vi "Filter Linearity Results.vi"(8 "error in (no error)":errorcluster, 10 "SensorID":i32, 11 "Linearity Results":T1[](array[typedef])) -> (0 "error out":errorcluster, 3 "Filtered Linearity Results":T1[](array[typedef]))   [LabVIEW 2026, in "Analysis.lvlib"]
uses:
  Analysis.lvlib
  Linearity Result.ctl
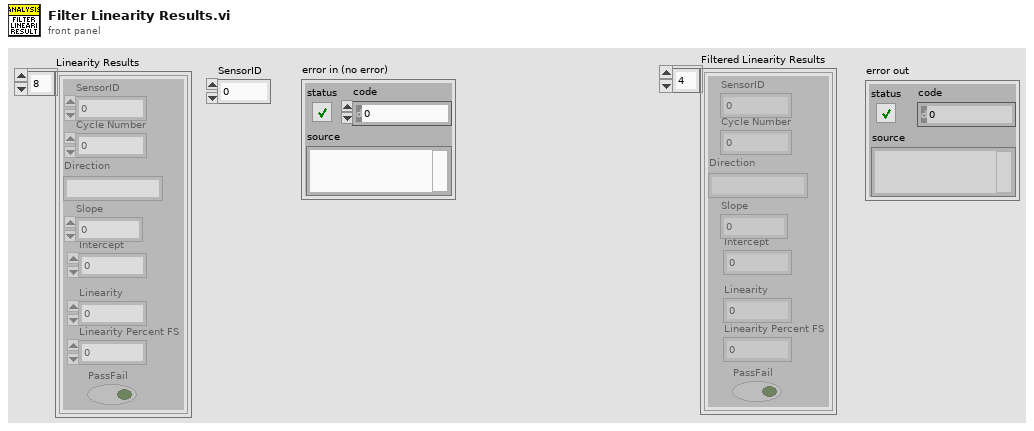
[diagram p1: front panel]
types:
  T1 = typedef "Analysis.lvlib/Linearity Result.ctl" = cluster{"Slope":dbl, "Intercept":dbl, "Cycle Number":i32, "SensorID":i32, "Linearity":dbl, "Linearity Percent FS":dbl, "Direction":string, "PassFail":bool}
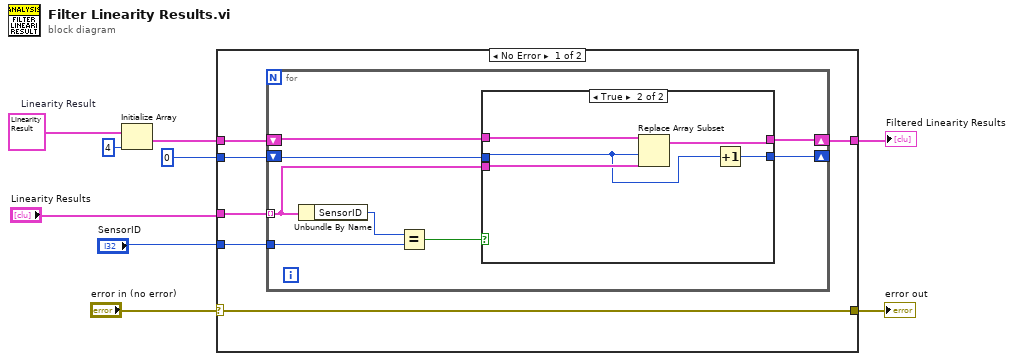
[diagram p0: block diagram]
diagram:
  w3 = T1 {"Slope"=1.0349176815530619, "Intercept"=2.9097848025003024, "Cycle Number"=0, "SensorID"=18, "Linearity"=2.9097848025003024, "Linearity Percent FS"=2.9097848025003024, "Direction"="Descending", "PassFail"=FALSE}  # Linearity Result
  n1 = Initialize Array(w3, 4 ("dimension size")) -> (w8:T1[])
  n2 = case shown="No Error" "error in (no error)" {
    selector: "error in (no error)" -> [w10 w32]
    tunnel: "SensorID" -> [w15 _]
    tunnel: "Linearity Results" -> [w14 _]
    tunnel: [w13 w31] -> w2
    tunnel: w8 -> [w12 w31]
    tunnel: 0 -> [w11 _]
    tunnel: [w10 w32] -> w4
    frame No Error {
      n3 = for {
        tunnel: w14 -> [w20] mode=indexing
        tunnel: w15 -> [w22]
        shift-right: [w18] -> w13
        shift-left: w12 -> [w19]
        shift-right: [w16] -> _
        shift-left: w11 -> [w17]
        n4 = Unbundle By Name(w20) -> ("SensorID"=w23:i32)
        n5 = Equal?(x=w23, y=w22) -> (x = y?=w21:bool)
        n6 = case shown="True" w21 {
          tunnel: w20 -> [_ w28]
          tunnel: w19 -> [w25 w30]
          tunnel: [w25 w29] -> w18
          tunnel: w17 -> [w24 w27]
          tunnel: [w24 w26] -> w16
          frame False {
          }
          frame True {
            n7 = Replace Array Subset(array=w30, new element=w28, index=w27) -> (w29:T1[])
            n8 = Increment(x=w27) -> (x+1=w26:i32)
          }
        }
      }
    }
    frame Error {
    }
  }
  "error out" <- w4
  "Filtered Linearity Results" <- w2
